vi "SoC2.vi"(3 "Coefficients":dbl[](array[numeric]), 4 "Time":i32, 5 "BAT Current (A)":dbl) -> (0 "Time (min)":i32, 1 "State":string, 2 "SoC (%)":i32)   [LabVIEW 2015]
uses:
  <vilib>/Analysis/polynomials.llb/Polynomial Roots (DBL).vi
  <vilib>/Analysis/NI_AALPro.lvlib
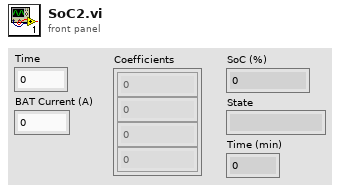
[diagram p1: front panel]
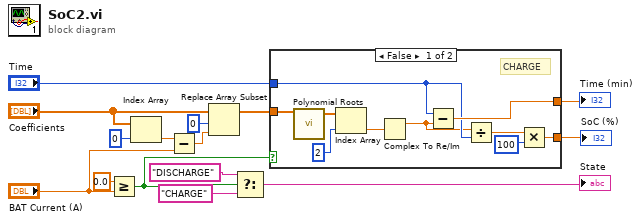
[diagram p0: block diagram]
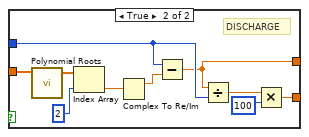
[diagram p2: hidden frame]
diagram:
  n1 = Greater Or Equal?(x=0.0, y="BAT Current (A)") -> (x >= y?=w12:bool)
  n2 = Index Array(array="Coefficients", index=0) -> (element=w6:dbl)
  n3 = Subtract(x=w6, y="BAT Current (A)") -> (x-y=w2:dbl)
  n4 = Replace Array Subset(array="Coefficients", new element=w2, index=0) -> (w1:dbl[])
  n5 = Select(t="DISCHARGE" ("f"), s=w12, f="CHARGE" ("t")) -> (s? t:f=→"State":string)
  n6 = case shown="False" w12 {
    tunnel: [w22 w27] -> w9
    tunnel: [w21 w33] -> w10
    tunnel: w1 -> [w20 w32]
    tunnel: "Time" -> [w19 w31]
    frame False {
      # "CHARGE"
      n7 = call-poly <vilib>:"Polynomial Roots.vi"("P(x)"=w20) -> ("Roots"=w16:cdb[])  [unwired: 9 in, 1 out]
      n8 = Index Array(array=w16, index=2) -> (element=w18:cdb)
      n9 = Complex To Re/Im(x + iy=w18) -> (x=w17:dbl)  [unwired: 1 out]
      n10 = Subtract(x=w19, y=w17) -> (x-y=w22:dbl)
      n11 = Divide(x=w17, y=w19) -> (x/y=w25:dbl)
      n12 = Multiply(x=w25, y=100) -> (x*y=w21:dbl)
    }
    frame True {
      # "DISCHARGE"
      n13 = call-poly <vilib>:"Polynomial Roots.vi"("P(x)"=w32) -> ("Roots"=w28:cdb[])  [unwired: 9 in, 1 out]
      n14 = Index Array(array=w28, index=2) -> (element=w30:cdb)
      n15 = Complex To Re/Im(x + iy=w30) -> (x=w29:dbl)  [unwired: 1 out]
      n16 = Subtract(x=w31, y=w29) -> (x-y=w27:dbl)
      n17 = Divide(x=w27, y=w31) -> (x/y=w35:dbl)
      n18 = Multiply(x=w35, y=100) -> (x*y=w33:dbl)
    }
  }
  "Time (min)" <- w9
  "SoC (%)" <- w10
